vi "Serve Buffer to Connection.vi"(7 "framework period":u32 format="%d us", 8 "error in":errorcluster, 9 "status":refnum<class "Status Pointer.lvclass">, 10 "buffer":refnum<class "Buffer.lvclass">, 11 "connection ID in":refnum<k5>) -> (0 "error out":errorcluster, 3 "connection ID out":refnum<k5>)   [LabVIEW 2019, in "DSF Core.lvlib" / "Data Server Thread.lvclass"]
uses:
  Data Server Thread.lvclass
  Buffer/Buffer.lvclass
  C:/Program Files (x86)/National Instruments/LabVIEW 2019/vi.lib/NI/Memory Manager/Classes/Pointer/Pointer.lvclass
  Status/Status Pointer.lvclass
  <vilib>/NI/Memory Manager/Classes/Pointer/Pointer.lvclass/Pointer.ctl
  Metrics.ctl
  <vilib>/NI/Memory Manager/Classes/Pointer/Get Address.vi
  <vilib>/NI/Memory Manager/Classes/Pointer/Get Size.vi
  <vilib>/NI/Memory Manager/Classes/Pointer/Read.vi
  <vilib>/NI/Memory Manager/Classes/Pointer/Read 1D U8.vi
  <vilib>/NI/Memory Manager/Classes/Pointer/Check Size.vi
  Status/Status Size.vi
  <vilib>/NI/Memory Manager/Classes/Pointer/Check Null Pointer.vi
  <vilib>/NI/Memory Manager/Classes/Pointer/Read (No Check).vi
  <vilib>/NI/Memory Manager/Classes/Pointer/Read (No Check) 1D U8.vi
  <vilib>/NI/Memory Manager/Classes/Pointer/Check Move.vi
  <vilib>/NI/Memory Manager/Classes/Pointer/Errors.vi
  <vilib>/NI/Memory Manager/Classes/Pointer/Out of Bounds.vi
  <vilib>/NI/Memory Manager/Classes/Pointer/Null Pointer.vi
  <vilib>/NI/Memory Manager/Classes/Pointer/Check Count.vi
  <vilib>/NI/Memory Manager/Classes/Pointer/Check Bounds (Power of 2).vi
  <vilib>/NI/Memory Manager/VIs/Write String to Source.vi
  <vilib>/NI/Memory Manager/Classes/Pointer/Write Pointer Size to Error.vi
  <vilib>/NI/Memory Manager/Classes/Pointer/Create Error.vi
  <vilib>/NI/Memory Manager/VIs/Write Numeric to Source.vi
  <vilib>/NI/Memory Manager/VIs/Write Numeric Scalar to Source (Base10 U64).vi
  <vilib>/NI/Memory Manager/Classes/Pointer/Check Bounds.vi
  <vilib>/NI/Memory Manager/VIs/New Error Cluster.vi
  <vilib>/NI/Memory Manager/VIs/New Error Cluster (512B).vi
  <vilib>/NI/Memory Manager/VIs/Set Error Status.vi
  <vilib>/NI/Memory Manager/VIs/Set Error Code.vi
  <vilib>/NI/Memory Manager/VIs/Set Error Source.vi
  <vilib>/NI/Memory Manager/Constants/Constants.vi
  <vilib>/NI/Memory Manager/Constants/Library Name.vi
  <vilib>/NI/Memory Manager/Classes/Pointer/Pointer Error Info.vi
  <vilib>/NI/Memory Manager/Constants/Pointer Class Name.vi
  <vilib>/NI/Memory Manager/Classes/Pointer/Check Bounds (Pointer).vi
  <vilib>/NI/Memory Manager/Classes/Pointer/Check Bounds (Buffer).vi
  <vilib>/NI/Memory Manager/Classes/Pointer/Buffer Underflow.vi
  <vilib>/NI/Memory Manager/Classes/Pointer/Pointer.lvclass
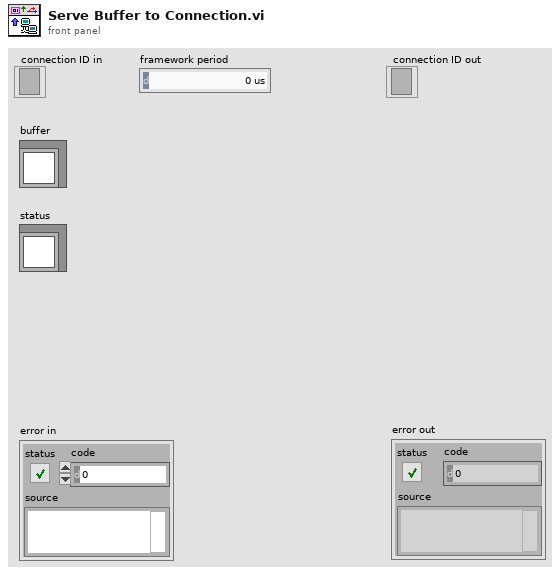
[diagram p1: front panel]
types:
  T1 = enum16{"big-endian, network order", "native, host order", "little-endian"}
  T2 = typedef "DSF Core.lvlib/Data Server Thread.lvclass/Metrics.ctl" = cluster{"framework period":u32, "iteration":u64, "late count":u64, "duration":u64}
  T3 = typedef "DSF Core.lvlib/Status Pointer.lvclass/Status Data.ctl" = cluster{"duration":u64, "period":u64, "iteration":u64, "late count":u64}
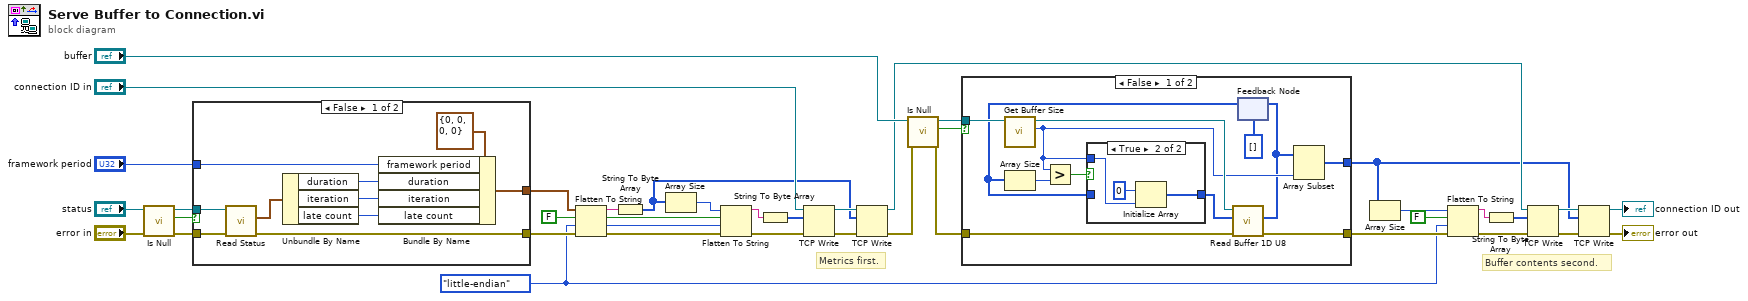
[diagram p0: block diagram]
diagram:
  w1 = T1."little-endian" ("byte order (0:big-endian, network order)")
  w25 = FALSE ("prepend array or string size? (T)")
  # "Buffer contents second."
  # "Metrics first."
  n1 = call <vilib>:"Is Null.vi"("error in (no error)"="error in", "Pointer in"="status") -> ("error out"=w32:errorcluster, "null?"=w31:bool, "Pointer out"=w30:refnum<class "Status Pointer.lvclass">)  [unwired: 7 in]
  n2 = case shown="False" w31 {
    tunnel: w32 -> [w46 w48]
    tunnel: w30 -> [w47 _]
    tunnel: [w42 w48] -> w21
    tunnel: "framework period" -> [w39 _]
    tunnel: [w41 _] -> w19
    frame False {
      n3 = call "Read Status.vi"("error in (no error)"=w46, "status pointer in"=w47) -> ("error out"=w42:errorcluster, "status"=w45:T3)  [unwired: 7 in, 1 out]
      n4 = Unbundle By Name(w45) -> ("duration"=w38:u64, "iteration"=w44:u64, "late count"=w43:u64)
      n5 = Bundle By Name(cluster=T2 {"framework period"=0, "iteration"=0, "late count"=0, "duration"=0} ("metrics"), "framework period"=w39, "duration"=w38, "iteration"=w44, "late count"=w43) -> (w41:T2)
    }
    frame True {
    }
  }
  n6 = Flatten To String(anything=w19, prepend array or string size? (T)=w25, byte order (0:big-endian, network order)=w1, error in (no error)=w21) -> (data string=w17:string, error out=w26:errorcluster)  [unwired: 1 out]
  n7 = String To Byte Array(string=w17) -> (unsigned byte array=w4:u8[])
  n8 = Array Size(array=w4) -> (size(s)=w24:i32)
  n9 = Flatten To String(anything=w24, prepend array or string size? (T)=w25, byte order (0:big-endian, network order)=w1, error in (no error)=w26) -> (data string=w3:string, error out=w23:errorcluster)  [unwired: 1 out]
  n10 = String To Byte Array(string=w3) -> (unsigned byte array=w2:u8[])
  n11 = TCP Write(connection ID="connection ID in", data in=w2, error in (no error)=w23) -> (connection ID out=w27:refnum<k5>, error out=w28:errorcluster)  [unwired: 1 in, 1 out]
  n12 = TCP Write(connection ID=w27, data in=w4, error in (no error)=w28) -> (connection ID out=w8:refnum<k5>, error out=w20:errorcluster)  [unwired: 1 in, 1 out]
  n13 = call <vilib>:"Is Null.vi"("error in (no error)"=w20, "Pointer in"="buffer") -> ("error out"=w36:errorcluster, "null?"=w35:bool, "Pointer out"=w37:refnum<class "Buffer.lvclass">)  [unwired: 7 in]
  n14 = case shown="False" w35 {
    tunnel: [w51 w65] -> w11
    tunnel: w37 -> [w55 _]
    tunnel: w36 -> [w54 w65]
    tunnel: [w49 _] -> w7
    frame False {
      n15 = call "Get Buffer Size.vi"("Buffer in"=w55) -> ("buffer size"=w52:u64, "Buffer out"=w56:refnum<class "Buffer.lvclass">)  [unwired: 9 in]
      n16 = feedback #1(u8[] []) -> (w53:u8[])
      n17 = Array Size(array=w53) -> (size(s)=w59:i32)
      n18 = Greater?(x=w52, y=w59) -> (0:w58:bool)
      n19 = case shown="True" w58 {
        tunnel: [w61 w63] -> w57
        tunnel: w53 -> [w61 _]
        tunnel: w52 -> [_ w62]
        frame False {
        }
        frame True {
          n20 = Initialize Array(u8 0, w62) -> (w63:u8[])
        }
      }
      n21 = call "Read Buffer 1D U8.vi"("error in (no error)"=w54, "dst array in"=w57, "Buffer in"=w56) -> ("error out"=w51:errorcluster, "dst array out"=w50:u8[])  [unwired: 5 in, 2 out]
      n22 = feedback-in #1(w50) -> ()
      n23 = Array Subset(array=w50, length=w52) -> (w49:u8[])  [unwired: 1 in]
    }
    frame True {
    }
  }
  n24 = Array Size(array=w7) -> (size(s)=w14:i32)
  n25 = Flatten To String(anything=w14, prepend array or string size? (T)=FALSE, byte order (0:big-endian, network order)=w1, error in (no error)=w11) -> (data string=w6:string, error out=w13:errorcluster)  [unwired: 1 out]
  n26 = String To Byte Array(string=w6) -> (unsigned byte array=w5:u8[])
  n27 = TCP Write(connection ID=w8, data in=w5, error in (no error)=w13) -> (connection ID out=w15:refnum<k5>, error out=w16:errorcluster)  [unwired: 1 in, 1 out]
  n28 = TCP Write(connection ID=w15, data in=w7, error in (no error)=w16) -> (connection ID out=→"connection ID out":refnum<k5>, error out=→"error out":errorcluster)  [unwired: 1 in, 1 out]
